vi "Salvar_excel.vi"(9 "Array":dbl[](array[numeric]), 11 "Filename":path=path "test.xlsx") -> ()   [LabVIEW 2019]
uses:
  <vilib>/express/express shared/transition.llb/Dynamic To Waveform Array.vi
  <vilib>/express/express signal manip/GetorSetDDTAttributes/Set DDT Attributes/SetT0.vi
  <vilib>/express/express shared/transition.llb/Waveform Array To Dynamic.vi
  <vilib>/express/express signal manip/GetorSetDDTAttributes/Set DDT Attributes/Set DDT Properties.xnode
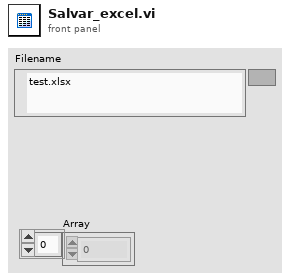
[diagram p1: front panel]
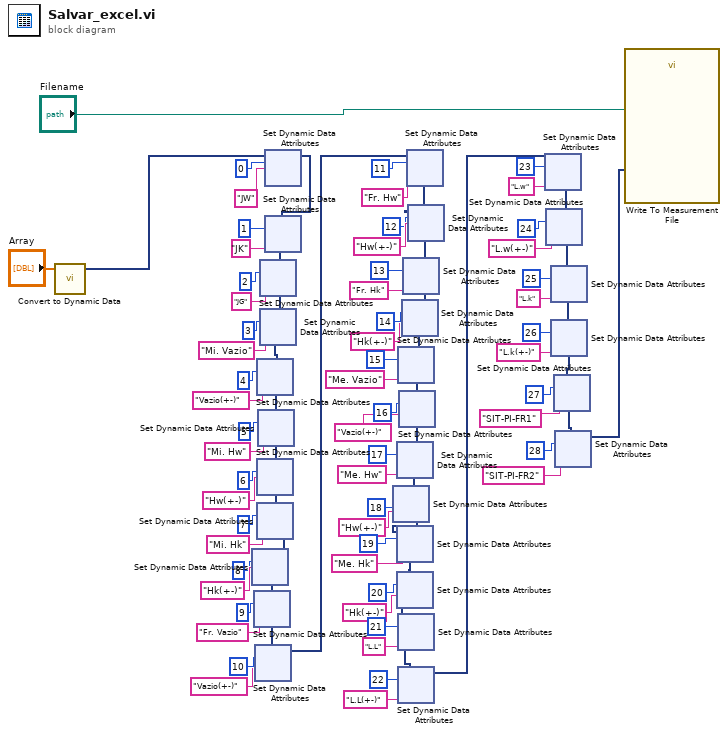
[diagram p0: block diagram]
diagram:
  n1 = call "Convert to Dynamic Data"("Array"="Array") -> ("Dynamic Data Type"=w2:dynamicdata)  [unwired: 3 in]
  n2 = xnode ("Set Dynamic Data Attributes")("Signals In"=w2, "Signal Index"=0, "Signal Name"="JW") -> ("Signals Out"=w64:dynamicdata)  [unwired: 1 in, 1 out]
  n3 = xnode ("Set Dynamic Data Attributes")("Signals In"=w64, "Signal Index"=1, "Signal Name"="JK") -> ("Signals Out"=w63:dynamicdata)  [unwired: 1 in, 1 out]
  n4 = xnode ("Set Dynamic Data Attributes")("Signals In"=w63, "Signal Index"=2, "Signal Name"="JG") -> ("Signals Out"=w62:dynamicdata)  [unwired: 1 in, 1 out]
  n5 = xnode ("Set Dynamic Data Attributes")("Signals In"=w62, "Signal Index"=3, "Signal Name"="Mi. Vazio") -> ("Signals Out"=w36:dynamicdata)  [unwired: 1 in, 1 out]
  n6 = xnode ("Set Dynamic Data Attributes")("Signals In"=w36, "Signal Index"=4, "Signal Name"="Vazio(+-)") -> ("Signals Out"=w19:dynamicdata)  [unwired: 1 in, 1 out]
  n7 = xnode ("Set Dynamic Data Attributes")("Signals In"=w19, "Signal Index"=5, "Signal Name"="Mi. Hw") -> ("Signals Out"=w18:dynamicdata)  [unwired: 1 in, 1 out]
  n8 = xnode ("Set Dynamic Data Attributes")("Signals In"=w18, "Signal Index"=6, "Signal Name"="Hw(+-)") -> ("Signals Out"=w17:dynamicdata)  [unwired: 1 in, 1 out]
  n9 = xnode ("Set Dynamic Data Attributes")("Signals In"=w17, "Signal Index"=7, "Signal Name"="Mi. Hk") -> ("Signals Out"=w16:dynamicdata)  [unwired: 1 in, 1 out]
  n10 = xnode ("Set Dynamic Data Attributes")("Signals In"=w16, "Signal Index"=8, "Signal Name"="Hk(+-)") -> ("Signals Out"=w15:dynamicdata)  [unwired: 1 in, 1 out]
  n11 = xnode ("Set Dynamic Data Attributes")("Signals In"=w15, "Signal Index"=9, "Signal Name"="Fr. Vazio") -> ("Signals Out"=w14:dynamicdata)  [unwired: 1 in, 1 out]
  n12 = xnode ("Set Dynamic Data Attributes")("Signals In"=w14, "Signal Index"=10, "Signal Name"="Vazio(+-)") -> ("Signals Out"=w13:dynamicdata)  [unwired: 1 in, 1 out]
  n13 = xnode ("Set Dynamic Data Attributes")("Signals In"=w13, "Signal Index"=11, "Signal Name"="Fr. Hw") -> ("Signals Out"=w12:dynamicdata)  [unwired: 1 in, 1 out]
  n14 = xnode ("Set Dynamic Data Attributes")("Signals In"=w12, "Signal Index"=12, "Signal Name"="Hw(+-)") -> ("Signals Out"=w11:dynamicdata)  [unwired: 1 in, 1 out]
  n15 = xnode ("Set Dynamic Data Attributes")("Signals In"=w11, "Signal Index"=13, "Signal Name"="Fr. Hk") -> ("Signals Out"=w10:dynamicdata)  [unwired: 1 in, 1 out]
  n16 = xnode ("Set Dynamic Data Attributes")("Signals In"=w10, "Signal Index"=14, "Signal Name"="Hk(+-)") -> ("Signals Out"=w9:dynamicdata)  [unwired: 1 in, 1 out]
  n17 = xnode ("Set Dynamic Data Attributes")("Signals In"=w9, "Signal Index"=15, "Signal Name"="Me. Vazio") -> ("Signals Out"=w8:dynamicdata)  [unwired: 1 in, 1 out]
  n18 = xnode ("Set Dynamic Data Attributes")("Signals In"=w8, "Signal Index"=16, "Signal Name"="Vazio(+-)") -> ("Signals Out"=w7:dynamicdata)  [unwired: 1 in, 1 out]
  n19 = xnode ("Set Dynamic Data Attributes")("Signals In"=w7, "Signal Index"=17, "Signal Name"="Me. Hw") -> ("Signals Out"=w6:dynamicdata)  [unwired: 1 in, 1 out]
  n20 = xnode ("Set Dynamic Data Attributes")("Signals In"=w6, "Signal Index"=18, "Signal Name"="Hw(+-)") -> ("Signals Out"=w20:dynamicdata)  [unwired: 1 in, 1 out]
  n21 = xnode ("Set Dynamic Data Attributes")("Signals In"=w20, "Signal Index"=19, "Signal Name"="Me. Hk") -> ("Signals Out"=w21:dynamicdata)  [unwired: 1 in, 1 out]
  n22 = xnode ("Set Dynamic Data Attributes")("Signals In"=w21, "Signal Index"=20, "Signal Name"="Hk(+-)") -> ("Signals Out"=w22:dynamicdata)  [unwired: 1 in, 1 out]
  n23 = xnode ("Set Dynamic Data Attributes")("Signals In"=w22, "Signal Index"=21, "Signal Name"="L.L") -> ("Signals Out"=w46:dynamicdata)  [unwired: 1 in, 1 out]
  n24 = xnode ("Set Dynamic Data Attributes")("Signals In"=w46, "Signal Index"=22, "Signal Name"="L.L(+-)") -> ("Signals Out"=w45:dynamicdata)  [unwired: 1 in, 1 out]
  n25 = xnode ("Set Dynamic Data Attributes")("Signals In"=w45, "Signal Index"=23, "Signal Name"="L.w") -> ("Signals Out"=w44:dynamicdata)  [unwired: 1 in, 1 out]
  n26 = xnode ("Set Dynamic Data Attributes")("Signals In"=w44, "Signal Index"=24, "Signal Name"="L.w(+-)") -> ("Signals Out"=w43:dynamicdata)  [unwired: 1 in, 1 out]
  n27 = xnode ("Set Dynamic Data Attributes")("Signals In"=w43, "Signal Index"=25, "Signal Name"="L.k") -> ("Signals Out"=w42:dynamicdata)  [unwired: 1 in, 1 out]
  n28 = xnode ("Set Dynamic Data Attributes")("Signals In"=w42, "Signal Index"=26, "Signal Name"="L.k(+-)") -> ("Signals Out"=w41:dynamicdata)  [unwired: 1 in, 1 out]
  n29 = xnode ("Set Dynamic Data Attributes")("Signals In"=w41, "Signal Index"=27, "Signal Name"="SIT-PI-FR1") -> ("Signals Out"=w56:dynamicdata)  [unwired: 1 in, 1 out]
  n30 = xnode ("Set Dynamic Data Attributes")("Signals In"=w56, "Signal Index"=28, "Signal Name"="SIT-PI-FR2") -> ("Signals Out"=w40:dynamicdata)  [unwired: 1 in, 1 out]
  n31 = call "Write To Measurement File"("Signals"=w40, "Filename"="Filename") -> ()  [unwired: 15 in, 3 out]
